vi "MultiRun.vi"() -> ()   [LabVIEW 2012]
uses:
  <vilib>/addons/database/Connection.llb/DB Tools Open Connec (Path).vi
  <vilib>/Utility/file.llb/Read From Spreadsheet File (string).vi
  <vilib>/addons/database/NI_Database_API.lvlib
panel:
  out "element 2":string
  out "f 3":bool
  out "standard error 5":string
  out "error out 3":errorcluster
  out "element":string
  out "f 2":bool
  out "standard error 4":string
  out "error out":errorcluster
  out "error out 2":errorcluster
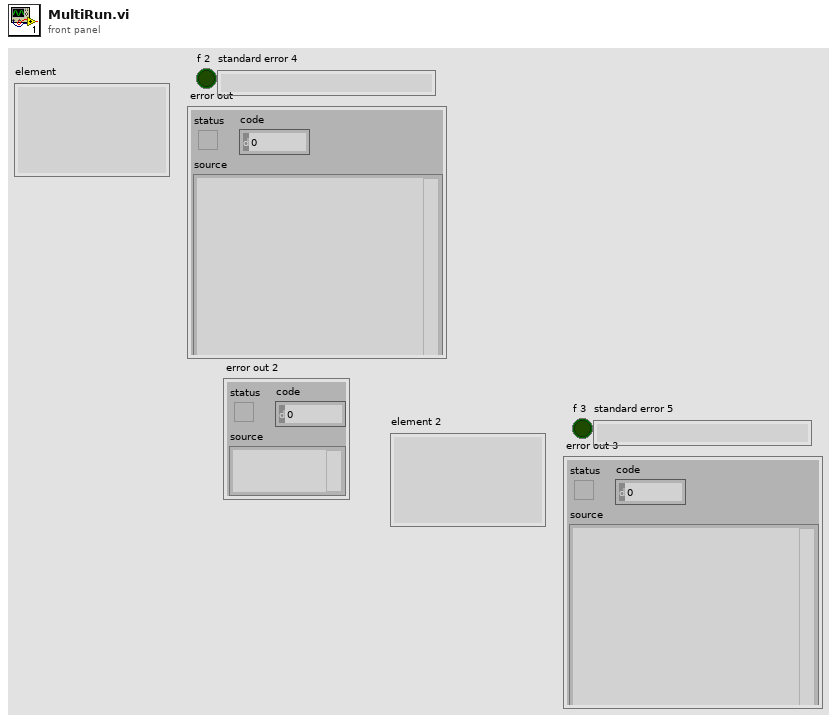
[diagram p1: front panel]
types:
  T1 = typedef "NI_Database_API.lvlib/Conn ObjectReference.ctl" = refnum<k1>
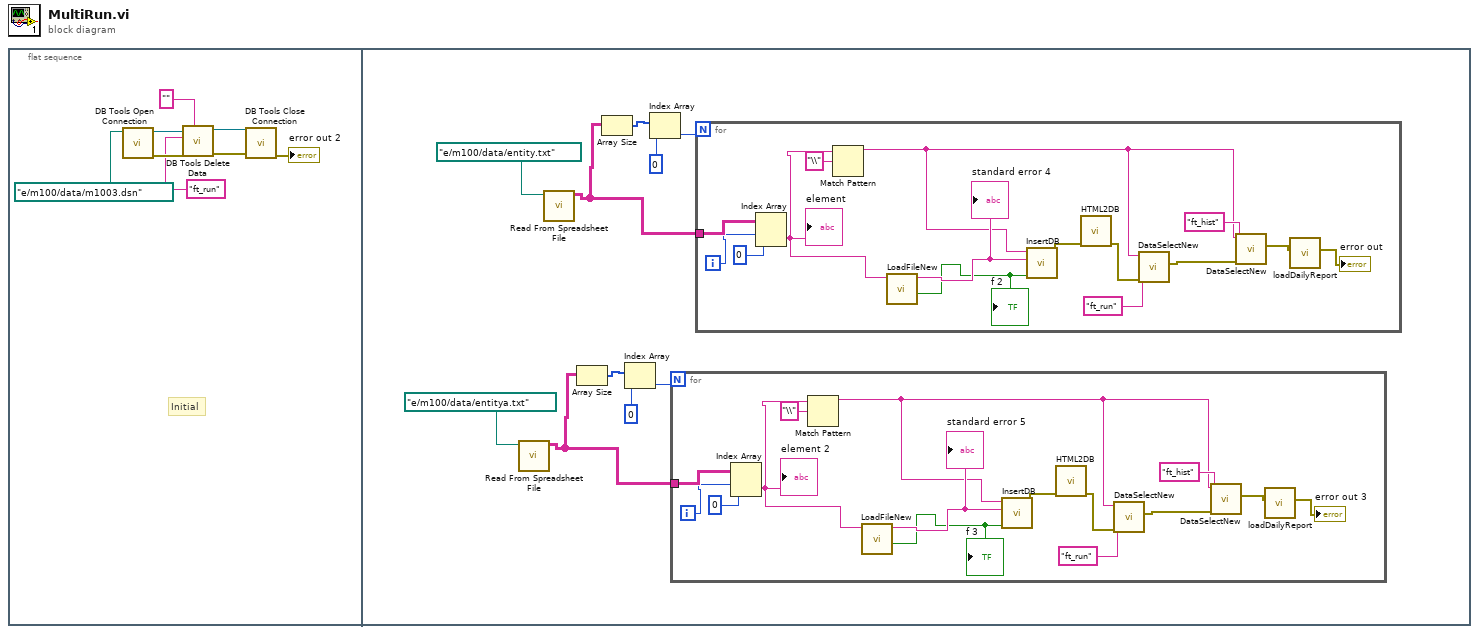
[diagram p0: block diagram]
diagram:
  n1 = flat-sequence {
    frame #0 {
      # "Initial"
      n2 = call-poly <vilib>:"DB Tools Open Connection.vi"("connection information"=path "e:/m100/data/m1003.dsn") -> ("error out"=w5:errorcluster, "connection reference"=w7:T1)  [unwired: 7 in]
      n3 = call <vilib>:"DB Tools Delete Data.vi"("condition"="", "error in (no error)"=w5, "table"="ft_run", "connection reference"=w7) -> ("error out"=w4:errorcluster, "connection reference out"=w6:T1)  [unwired: 6 in]
      n4 = call <vilib>:"DB Tools Close Connection.vi"("error in (no error)"=w4, "connection reference"=w6) -> ("error out"=→"error out 2":errorcluster)  [unwired: 5 in]
    }
    frame #1 {
      n5 = call-poly <vilib>:"Read From Spreadsheet File.vi"("file path (dialog if empty)"=path "e:/m100/data/entitya.txt" ("file path (use dialog)")) -> ("all rows"=w9:string[][])  [unwired: 6 in, 4 out]
      n6 = call-poly <vilib>:"Read From Spreadsheet File.vi"("file path (dialog if empty)"=path "e:/m100/data/entity.txt" ("file path (use dialog)")) -> ("all rows"=w14:string[][])  [unwired: 6 in, 4 out]
      n7 = Array Size(array=w9) -> (size(s)=w12:i32[])
      n8 = Array Size(array=w14) -> (size(s)=w17:i32[])
      n9 = Index Array(array=w12, index=0) -> (element=w10:i32)
      n10 = Index Array(array=w17, index=0) -> (element=w15:i32)
      n11 = for {
        N: w10 -> [_]
        tunnel: w9 -> [w33]
        i -> [w31]
        n12 = Index Array(array=w33, index (row)=w31, index (col)=0 ("disabled index (col)")) -> (element=w27:string)
        "element 2" <- w27
        n13 = Match Pattern(string=w27, regular expression="\\") -> (before substring=w21:string)  [unwired: 1 in, 3 out]
        n14 = call "LoadFileNew.vi"("folder"=w27) -> ("f"=w28:bool, "Lot"=w29:string)  [unwired: 9 in]
        "f 3" <- w28
        "standard error 5" <- w29
        n15 = call "InsertDB.vi"("Boolean"=w28, "String"=w29, "Entity"=w21) -> ("error out"=w26:errorcluster)  [unwired: 7 in]
        n16 = call "HTML2DB.vi"("error in (no error)"=w26) -> ("error out"=w25:errorcluster)  [unwired: 10 in]
        n17 = call "DataSelectNew.vi"("error in (no error)"=w25, "Table"="ft_run", "Machine"=w21) -> ("error out"=w23:errorcluster)  [unwired: 8 in]
        n18 = call "DataSelectNew.vi"("error in (no error)"=w23, "Table"="ft_hist", "Machine"=w21) -> ("error out"=w20:errorcluster)  [unwired: 8 in]
        n19 = call "loadDailyReport.vi"("error in (no error)"=w20) -> ("error out"=→"error out 3":errorcluster)  [unwired: 10 in]
      }
      n20 = for {
        N: w15 -> [_]
        tunnel: w14 -> [w48]
        i -> [w46]
        n21 = Index Array(array=w48, index (row)=w46, index (col)=0 ("disabled index (col)")) -> (element=w42:string)
        "element" <- w42
        n22 = Match Pattern(string=w42, regular expression="\\") -> (before substring=w36:string)  [unwired: 1 in, 3 out]
        n23 = call "LoadFileNew.vi"("folder"=w42) -> ("f"=w43:bool, "Lot"=w44:string)  [unwired: 9 in]
        "f 2" <- w43
        "standard error 4" <- w44
        n24 = call "InsertDB.vi"("Boolean"=w43, "String"=w44, "Entity"=w36) -> ("error out"=w41:errorcluster)  [unwired: 7 in]
        n25 = call "HTML2DB.vi"("error in (no error)"=w41) -> ("error out"=w40:errorcluster)  [unwired: 10 in]
        n26 = call "DataSelectNew.vi"("error in (no error)"=w40, "Table"="ft_run", "Machine"=w36) -> ("error out"=w38:errorcluster)  [unwired: 8 in]
        n27 = call "DataSelectNew.vi"("error in (no error)"=w38, "Table"="ft_hist", "Machine"=w36) -> ("error out"=w35:errorcluster)  [unwired: 8 in]
        n28 = call "loadDailyReport.vi"("error in (no error)"=w35) -> ("error out"=→"error out":errorcluster)  [unwired: 10 in]
      }
    }
  }
